vi "test.vi"(4 "length":i64, 5 "subvi cycle":refnum<vi>, 6 "sample array":i32[](array[numeric]), 7 "rand array sub":dbl[](array[numeric]), 8 "subvi timing":refnum<vi>, 9 "Graph Refnum":refnum<vi>, 10 "start time":ext format="%#_13g", 11 "rand array sub refnum":refnum<vi>) -> ()   [LabVIEW 2014]
panel:
  out "timing":dbl
  out "current sample":dbl format="%#_13g"
  out "previous sample":dbl format="%#_13g"
  out "rand array sub out":dbl[](array[numeric])
  out "sample number":i32
  out "rand plot sub":cluster{i32, "element":dbl}[](graph)
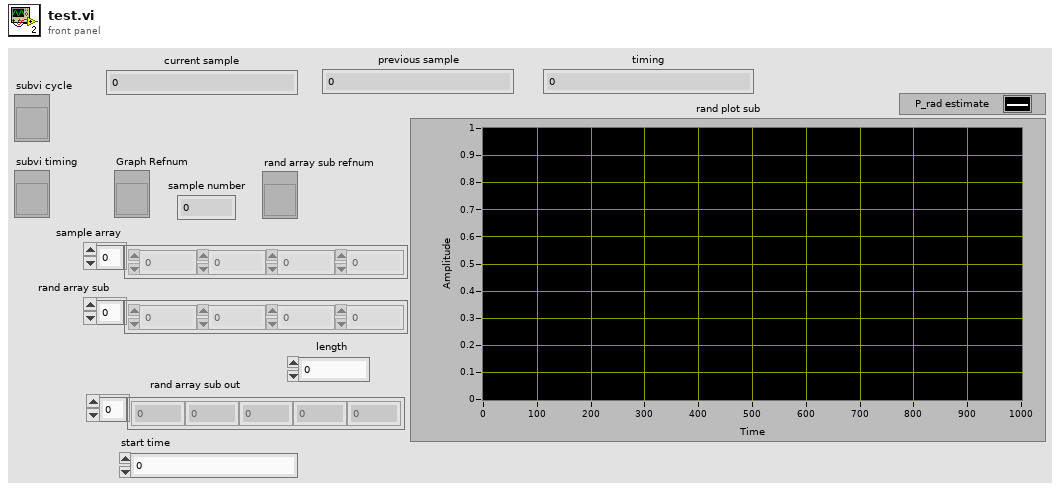
[diagram p1: front panel]
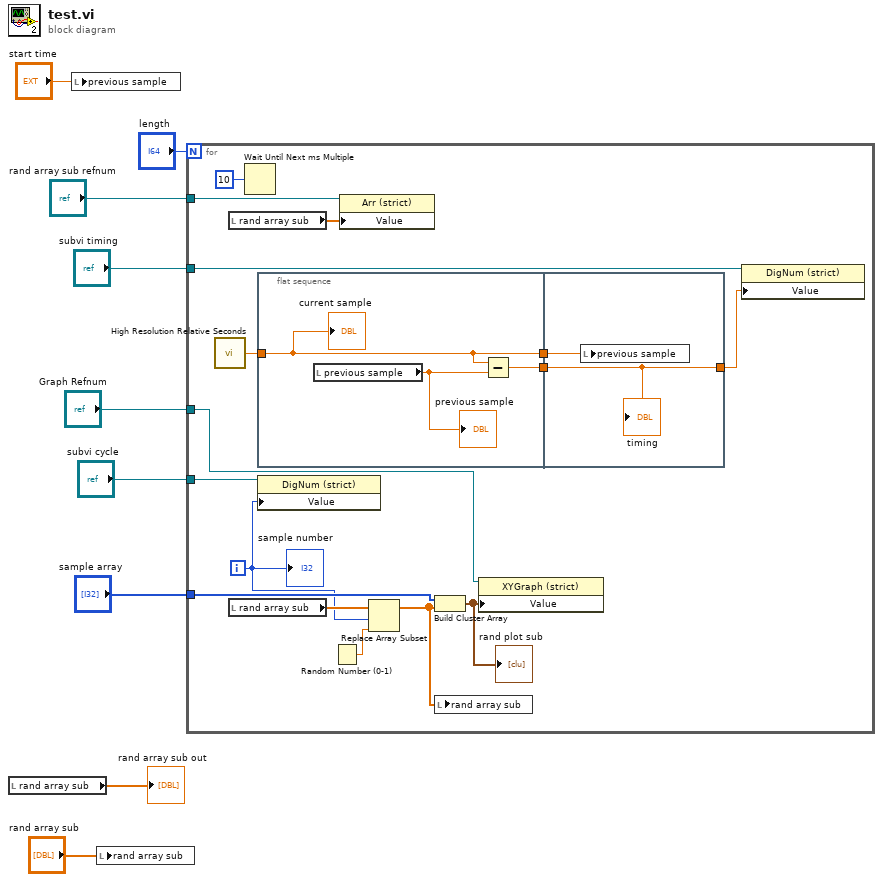
[diagram p0: block diagram]
diagram:
  n1 = local read "rand array sub"() -> (→"rand array sub out":dbl[])
  n2 = local write "previous sample"("start time") -> ()
  n3 = local write "rand array sub"("rand array sub") -> ()
  n4 = for {
    N: "length" -> [_]
    tunnel: "Graph Refnum" -> [w25]
    tunnel: "sample array" -> [w22]
    tunnel: "rand array sub refnum" -> [w18]
    tunnel: "subvi timing" -> [w13]
    tunnel: "subvi cycle" -> [w16]
    i -> [w15]
    n5 = call <vilib>:"High Resolution Relative Seconds.vi"() -> ("relative seconds"=w14:dbl)
    n6 = local read "rand array sub"() -> (w17:dbl[])
    n7 = local read "rand array sub"() -> (w20:dbl[])
    n8 = Wait Until Next ms Multiple(millisecond multiple=10) -> ()  [unwired: 1 out]
    n9 = flat-sequence {
      tunnel: w14 -> [w27]
      tunnel: [w27] -> w12
      tunnel: [w26] -> w11
      tunnel: w12 -> [w30]
      tunnel: w11 -> [w29]
      tunnel: [w29] -> w10
      frame #0 {
        n10 = local read "previous sample"() -> (w28:dbl)
        "previous sample" <- w28
        n11 = Subtract(x=w27, y=w28) -> (x-y=w26:dbl)
        "current sample" <- w27
      }
      frame #1 {
        n12 = local write "previous sample"(w30) -> ()
        "timing" <- w29
      }
    }
    n13 = property class="DigNum (strict)"(reference=w16, "Value"=w15) -> ()  [unwired: 1 in, 2 out]
    n14 = Random Number (0-1)() -> (number: 0 to 1=w23:dbl)
    n15 = property class="Arr (strict)"(reference=w18, "Value"=w17) -> ()  [unwired: 1 in, 2 out]
    n16 = Replace Array Subset(array=w20, new element=w23, index=w15) -> (w19:dbl[])
    n17 = Build Cluster Array(w22, w19) -> (w21:cluster{i32, "element":dbl}[])
    "rand plot sub" <- w21
    n18 = local write "rand array sub"(w19) -> ()
    n19 = property class="XYGraph (strict)"(reference=w25, "Value"=w21) -> ()  [unwired: 1 in, 2 out]
    n20 = property class="DigNum (strict)"(reference=w13, "Value"=w10) -> ()  [unwired: 1 in, 2 out]
    "sample number" <- w15
  }
